vi "AIsFIFORTTest.vi"() -> (0 "AIs":dbl[](array[numeric]))   [LabVIEW 2010]
uses:
  <vilib>/rvi/interface/nirviMethod/nirviMethod.xnode
  C:/Users/HAGAR-IV/Desktop/Zeugs/Johnny/pertrasgc fpga/FPGA-Programm-10-14.vi
  <vilib>/rvi/interface/nirviReadWriteControl/nirviReadWriteControl.xnode
  <vilib>/rvi/errors/niLvFpgaWhatHappensToTopLevelVI.ctl
  <vilib>/rvi/interface/common/niFpgaNodeNameForErrorReporting.ctl
  <vilib>/rvi/errors/niLvFpgaAdjustHostInterfaceError.vi
  C:/Users/HAGAR-IV/Desktop/Zeugs/markus/version feb 2012/FPGA Bitfiles/pertrasgcfpga2_FPGATarget_FPGA-Programm-10_16368CB6.lvbitx
  NiFpgaLv.dll
  <vilib>/Utility/error.llb/Error Cluster From Error Code.vi
  <vilib>/rvi/interface/nirviCloseFPGA/nirviCloseFPGA.xnode
  <vilib>/FPGAPlugInAG/cRIO-9114/niLvFpga_Close_cRIO-9114.vi
panel:
  out "Elements Remaining":u32
  out "Numerisch 2":i32
  out "Numerisch":dbl
  out "Array":dbl[](array[numeric])
  in  "Stop":bool
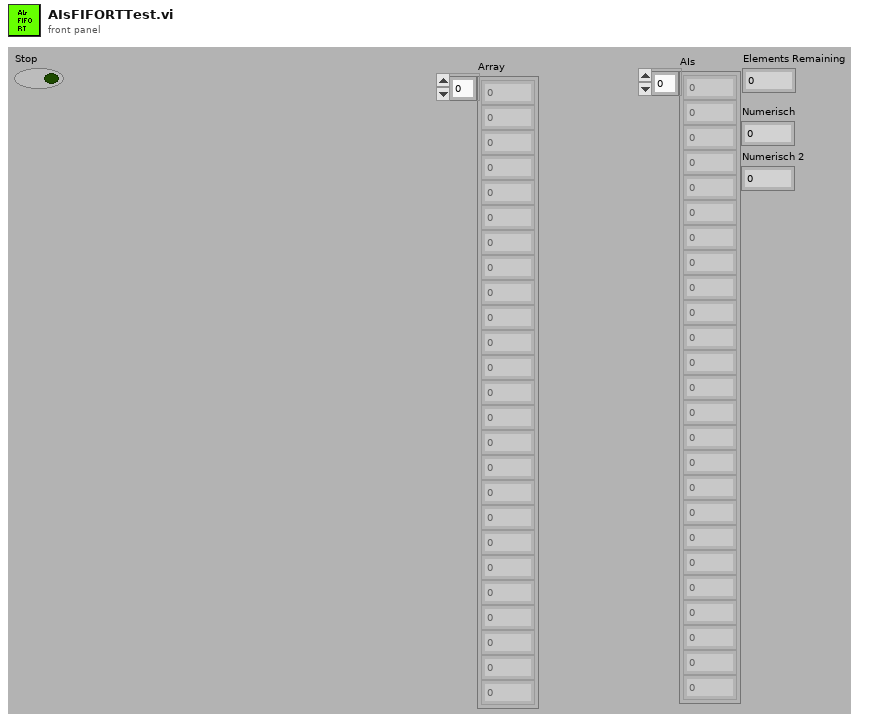
[diagram p1: front panel]
types:
  T1 = typedef "niFpgaNodeNameForErrorReporting.ctl" = enum16{"Open FPGA VI Reference", "Read/Write Control", "Invoke Method: Abort", "Invoke Method: Acknowledge IRQ", "Invoke Method: Download", "Invoke Method: FIFO.Configure", "Invoke Method: FIFO.Read", "Invoke Method: FIFO.Start", "Invoke Method: FIFO.Stop", "Invoke Method: FIFO.Write", "Invoke Method: Reset", "Invoke Method: Run", "Invoke Method: Wait on IRQ", "Close FPGA VI Reference"}
  T2 = typedef "niLvFpgaWhatHappensToTopLevelVI.ctl" = enum16{"top level VI scripted behind XNode", "top level VI inlined behind XNode"}
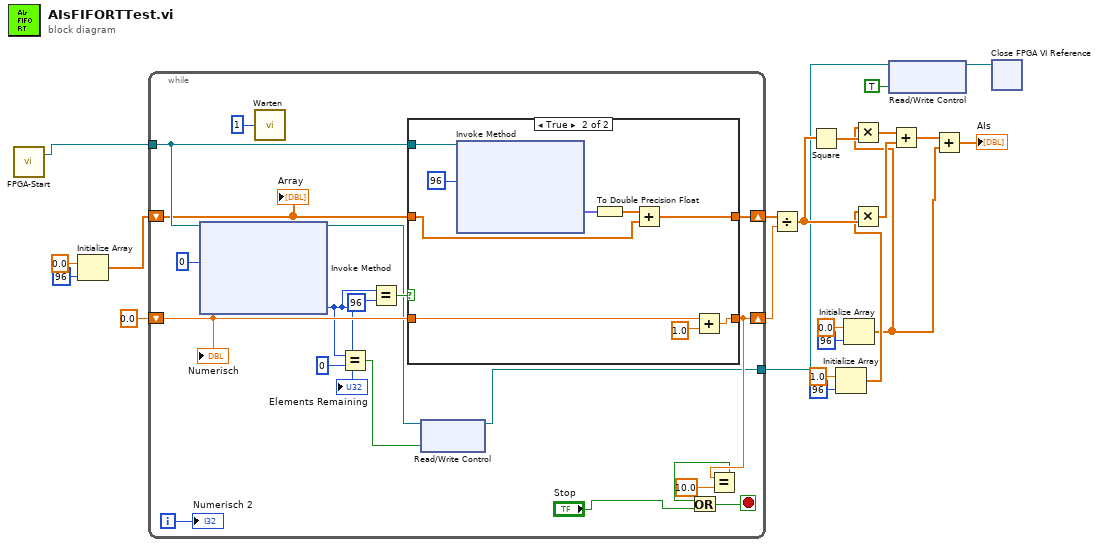
[diagram p0: block diagram]
diagram:
  n1 = call "FPGA-Start.vi"() -> ("FPGA VI Reference Out"=w10:refnum<k20>)  [unwired: 2 in, 1 out]
  n2 = Initialize Array(0.0 ("Element"), 96 ("Dimension")) -> (w13:dbl[])
  n3 = while {
    tunnel: w10 -> [w41]
    shift-right: [w35] -> w21
    shift-left: w13 -> [w36]
    shift-right: [w33] -> w12
    shift-left: 0.0 -> [w34]
    tunnel: [w25] -> w3
    i -> [w23]
    stop <- w26 stop-if-true
    n4 = xnode "Invoke Method"("FPGA VI Reference In"=w41, "Number of Elements"=u32 0) -> ("FPGA VI Reference Out"=w28:refnum<k20>, "Elements Remaining"=w31:u32)  [unwired: 2 in, 2 out]
    "Elements Remaining" <- w31
    n5 = call "Warten"("Count(mSec)"=u32 1) -> ()  [unwired: 1 out]
    n6 = Equal?(x=w31, y=u32 0) -> (x = y?=w29:bool)
    n7 = Equal?(x=w31, y=u32 96) -> (x = y?=w38:bool)
    n8 = case shown="True" w38 {
      tunnel: w41 -> [_ w162]
      tunnel: w36 -> [w153 w158]
      tunnel: [w153 w157] -> w35
      tunnel: w34 -> [w152 w156]
      tunnel: [w152 w154] -> w33
      frame False {
      }
      frame True {
        n9 = xnode "Invoke Method"("FPGA VI Reference In"=w162, "Number of Elements"=u32 96) -> ("Data"=w160:fxp<+/-,26,5>[])  [unwired: 2 in, 3 out]
        n10 = To Double Precision Float(number=w160) -> (double precision float=w159:dbl[])
        n11 = Add(x=w159, y=w158) -> (x+y=w157:dbl[])
        n12 = Add(x=w156, y=1.0) -> (x+y=w154:dbl)
      }
    }
    n13 = xnode "Read/Write Control"("FPGA VI Reference In"=w28, "FIFO leer"=w29) -> ("FPGA VI Reference Out"=w25:refnum<k20>)  [unwired: 1 in, 1 out]
    n14 = Equal?(x=w33, y=10.0) -> (x = y?=w27:bool)
    n15 = Or(x=w27, y="Stop") -> (x .or. y?=w26:bool)
    "Array" <- w36
    "Numerisch" <- w34
    "Numerisch 2" <- w23
  }
  n16 = Divide(x=w21, y=w12) -> (x/y=w19:dbl[])
  n17 = Square(x=w19) -> (x^2=w20:dbl[])
  n18 = Initialize Array(1.0 ("Element"), 96 ("Dimension")) -> (w5:dbl[])
  n19 = Initialize Array(0.0 ("Element"), 96 ("Dimension")) -> (w4:dbl[])
  n20 = Multiply(x=w4, y=w20) -> (x*y=w18:dbl[])
  n21 = Multiply(x=w5, y=w19) -> (x*y=w17:dbl[])
  n22 = xnode "Read/Write Control"("FPGA VI Reference In"=w3, "global stop"=TRUE) -> ("FPGA VI Reference Out"=w1:refnum<k20>)  [unwired: 1 in, 1 out]
  n23 = Add(x=w18, y=w17) -> (x+y=w16:dbl[])
  n24 = Add(x=w16, y=w4) -> (x+y=→"AIs":dbl[])
  n25 = xnode "Close FPGA VI Reference"("FPGA VI Reference In"=w1) -> ()  [unwired: 1 in, 1 out]
